vi "S4ACS_Controller.vi"() -> ()   [LabVIEW 2018]
uses:
  Channel Manager/Channel Manager.lvclass
  Channel Manager/Channel Manager.lvclass/Channel Manager.ctl
  Channel/Channel.lvclass
panel:
  out "Error":string
  in  "Stop Button":bool
  in  "Computer Specifier":u8=1
  out "Message:":string
  in  "Channel Manager.lvclass":refnum<class "Channel Manager.lvclass">
  # "SPARC4 - Acquisition Controler"
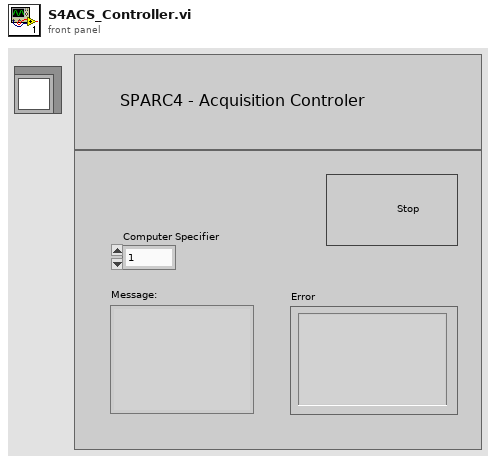
[diagram p1: front panel]
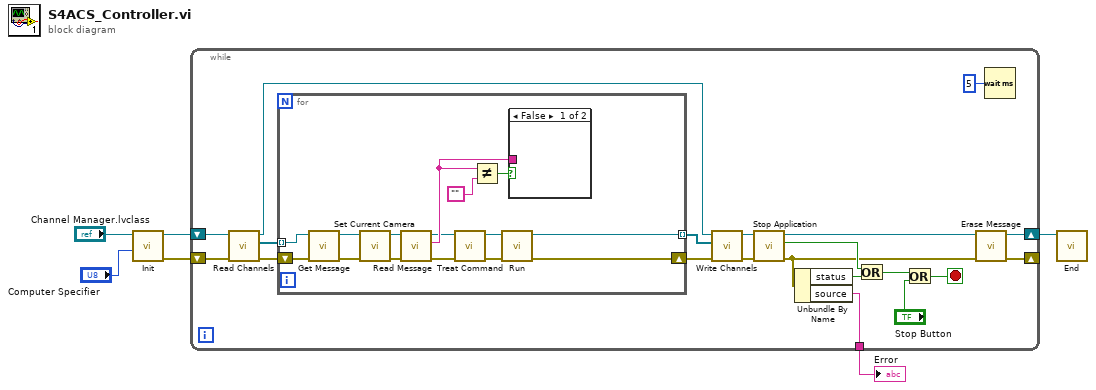
[diagram p0: block diagram]
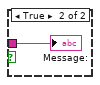
[diagram p2: hidden frame]
diagram:
  n1 = call "Init.vi"("Computer Specifier"="Computer Specifier", "Channel Manager in"="Channel Manager.lvclass") -> ("error out"=w5:errorcluster, "Channel Manager out"=w6:refnum<class "Channel Manager.lvclass">)  [unwired: 8 in]
  n2 = while {
    shift-right: [w16] -> _
    shift-left: w5 -> [w8]
    shift-right: [w14] -> w4
    shift-left: w6 -> [w9]
    tunnel: [w7] -> w1
    stop <- w10 stop-if-true
    n3 = call "Read Channels.vi"("error in (no error)"=w8, "Channel Manager in"=w9) -> ("error out"=w25:errorcluster, "Array"=w26:refnum<class "Channel.lvclass">[], "Channel Manager out"=w23:refnum<class "Channel Manager.lvclass">)  [unwired: 7 in]
    n4 = for {
      tunnel: w26 -> [w33] mode=indexing
      tunnel: [w40] -> w24 mode=indexing
      shift-right: [w41] -> w22
      shift-left: w25 -> [w34]
      n5 = call "Get Message.vi"("error in (no error)"=w34, "Channel in"=w33) -> ("error out"=w27:errorcluster, "Channel out"=w28:refnum<class "Channel.lvclass">)  [unwired: 8 in]
      n6 = call "Set Current Camera.vi"("error in (no error)"=w27, "Channel in"=w28) -> ("error out"=w36:errorcluster, "Channel out"=w35:refnum<class "Channel.lvclass">)  [unwired: 8 in]
      n7 = call "Read Message.vi"("error in (no error)"=w36, "Channel in"=w35) -> ("error out"=w30:errorcluster, "Message"=w37:string, "Channel out"=w31:refnum<class "Channel.lvclass">)  [unwired: 7 in]
      n8 = call "Treat Command.vi"("error in (no error)"=w30, "Channel in"=w31) -> ("error out"=w29:errorcluster, "Channel out"=w32:refnum<class "Channel.lvclass">)  [unwired: 8 in]
      n9 = Not Equal?(x=w37, y="") -> (x != y?=w38:bool)
      n10 = call "Run.vi"("error in (no error)"=w29, "Channel in"=w32) -> ("error out"=w41:errorcluster, "Channel out"=w40:refnum<class "Channel.lvclass">)  [unwired: 8 in]
      n11 = case shown="False" w38 {
        tunnel: w37 -> [_ w42]
        frame False {
        }
        frame True {
          "Message:" <- w42
        }
      }
    }
    n12 = call "Write Channels.vi"("error in (no error)"=w22, "Channels Array"=w24, "Channel Manager in"=w23) -> ("error out"=w21:errorcluster, "Channel Manager out"=w20:refnum<class "Channel Manager.lvclass">)  [unwired: 7 in]
    n13 = call "Stop Application.vi"("error in (no error)"=w21, "Channel Manager in"=w20) -> ("error out"=w15:errorcluster, "Stop Application"=w18:bool, "Channel Manager out"=w13:refnum<class "Channel Manager.lvclass">)  [unwired: 7 in]
    n14 = Unbundle By Name(w15) -> ("status"=w19:bool, "source"=w7:string)
    n15 = Or(x=w18, y=w19) -> (x .or. y?=w12:bool)
    n16 = Or(x=w12, y="Stop Button") -> (x .or. y?=w10:bool)
    n17 = call "Erase Message.vi"("error in (no error)"=w15, "Channel Manager in"=w13) -> ("error out"=w16:errorcluster, "Channel Manager out"=w14:refnum<class "Channel Manager.lvclass">)  [unwired: 8 in]
    n18 = Wait (ms)(milliseconds to wait=u32 5) -> ()  [unwired: 1 out]
  }
  "Error" <- w1
  n19 = call "End.vi"("Channel Manager in"=w4) -> ()  [unwired: 9 in, 2 out]
